vi "getReferenceTimeProtocol.vi"(8 "error in (no error)":errorcluster, 11 "IReferenceDomainInfo in":refnum<class "IReferenceDomainInfo.lvclass">) -> (0 "error out":errorcluster, 2 "TimeProtocol out":T1 items=["daqTimeProtocolUnknown", "daqTimeProtocolTai", "daqTimeProtocolGps", "daqTimeProtocolUtc"], 3 "IReferenceDomainInfo out":refnum<class "IReferenceDomainInfo.lvclass">)   [LabVIEW 2022 SP3, in "openDAQ.lvlib" / "IBaseObject.lvlib" / "IReferenceDomainInfo.lvlib" / "IReferenceDomainInfo.lvclass"]
uses:
  <instrlib>/openDAQ/Public/Classes/IReferenceDomainInfo/IReferenceDomainInfo.lvclass
  <instrlib>/openDAQ/Public/Classes/IReferenceDomainInfo/IReferenceDomainInfo.lvclass/IReferenceDomainInfo.ctl
  <instrlib>/openDAQ/Binaries/Windows/x86/copendaq32.dll
  <instrlib>/openDAQ/Public/TypeDef/daqTimeProtocol.ctl
  <instrlib>/openDAQ/openDAQ.lvlib
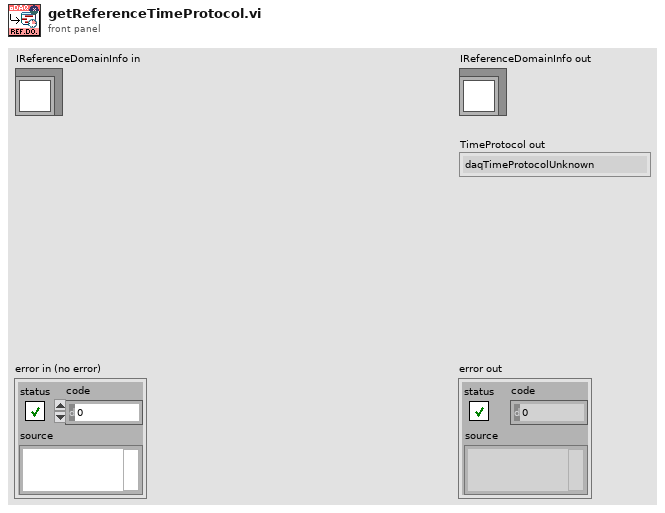
[diagram p1: front panel]
types:
  T1 = typedef "openDAQ.lvlib/daqTimeProtocol.ctl" = u16
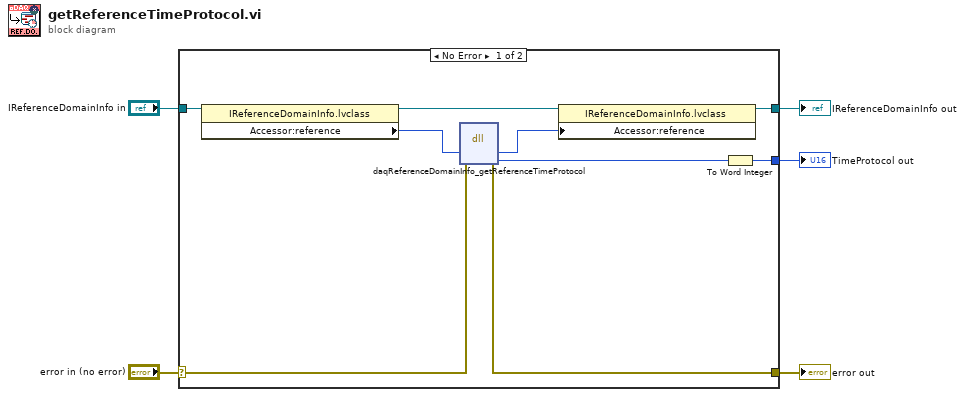
[diagram p0: block diagram]
diagram:
  n1 = case shown="No Error" "error in (no error)" {
    selector: "error in (no error)" -> [w13 w16]
    tunnel: [w12 w16] -> w4
    tunnel: [w7 w15] -> w2
    tunnel: "IReferenceDomainInfo in" -> [w14 w15]
    tunnel: [w9 _] -> w1
    frame No Error {
      n2 = property class="IReferenceDomainInfo.lvclass"(reference=w14) -> (reference out=w8:refnum<class "IReferenceDomainInfo.lvclass">, "Accessor:reference"=w11:i64)  [unwired: 1 in, 1 out]
      n3 = dll-call lib="C:/Program Files (x86)/National Instruments/LabVIEW 2022/instr.lib/openDAQ/Binaries/Windows/x86/copendaq*.*" fn="daqReferenceDomainInfo_getReferenceTimeProtocol"(error in=w13, "referenceDomainInfo"=w11) -> (error out=w12:errorcluster, "referenceDomainInfo"=w6:i64, "timeProtocol"=w10:i64)  [unwired: 4 in, 1 out]
      n4 = property class="IReferenceDomainInfo.lvclass"(reference=w8, "Accessor:reference"=w6) -> (reference out=w7:refnum<class "IReferenceDomainInfo.lvclass">)  [unwired: 1 in, 1 out]
      n5 = To Word Integer(number=w10) -> (16bit integer=w9:i16)
    }
    frame Error {
    }
  }
  "error out" <- w4
  "IReferenceDomainInfo out" <- w2
  "TimeProtocol out" <- w1
